vi "StepMotorStateMachine.vi"() -> ()   [LabVIEW 2011]
panel:
  in  "y":i32=360
  out "x-y*floor(x/y)":i32=173
  out "floor(x/y)":i32=148
  out "Diagrama Fasorial":picture
  out "Gauge":dbl(knob)=173.0 scale=0.0..360.0
  out "Counter":i32=53453
  in  "Direccion de Giro":bool=TRUE
  in  "stop":bool
  out "Array":bool[](array[boolean])=[TRUE, FALSE, TRUE, FALSE]
  out "Boolean array":bool[](array[boolean])=[FALSE, TRUE, FALSE, TRUE, FALSE, FALSE, FALSE, FALSE, FALSE, FALSE, FALSE, FALSE, FALSE, FALSE, FALSE, FALSE, FALSE, FALSE, FALSE, FALSE, FALSE, FALSE, FALSE, FALSE, FALSE, FALSE, FALSE, FALSE, FALSE, FALSE, FALSE, FALSE]
  out "Estado":u8=10
  in  "millisecond multiple 2":u32(knob) scale=0.0..300.0
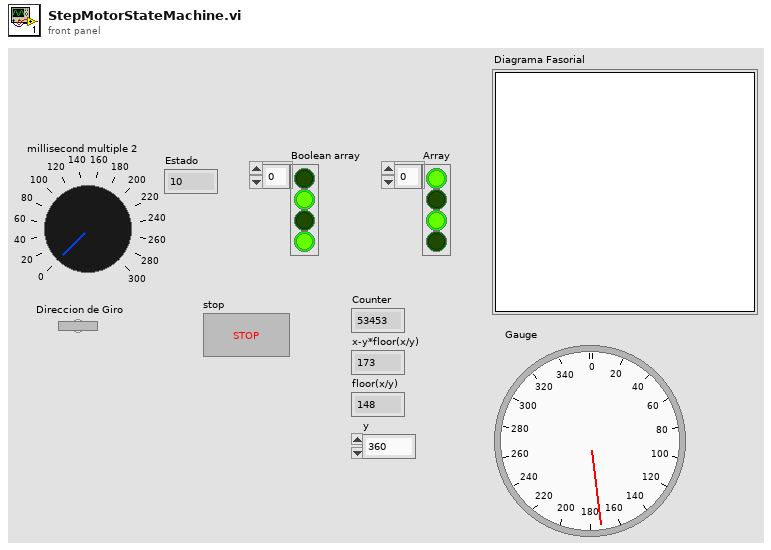
[diagram p1: front panel]
types:
  T1 = typedef "LVBoundsTypeDef.ctl" = cluster{"Width":u32, "Height":u32}
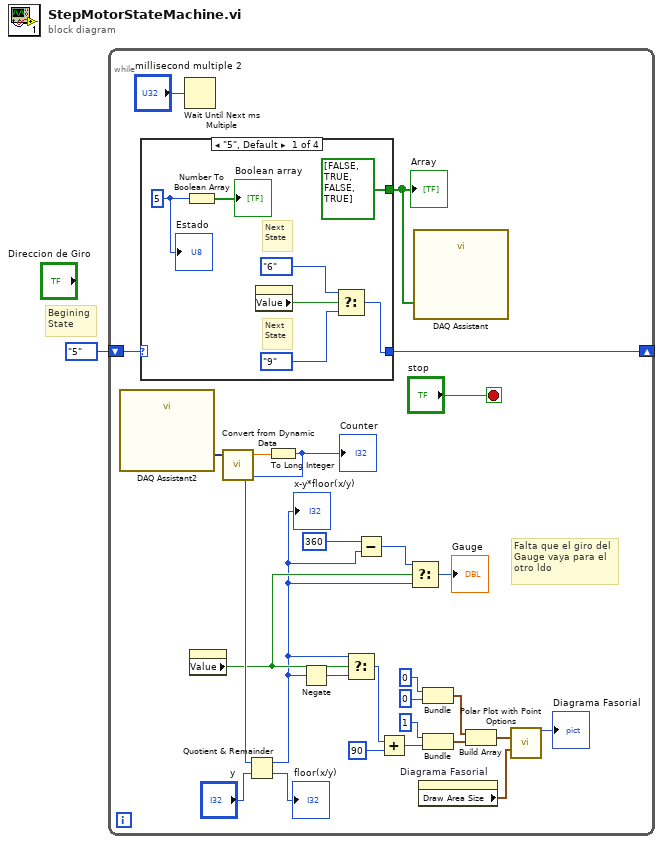
[diagram p0: block diagram]
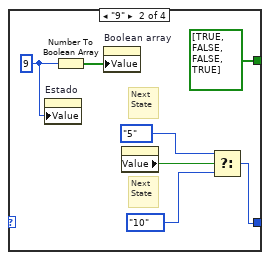
[diagram p2: hidden frame]
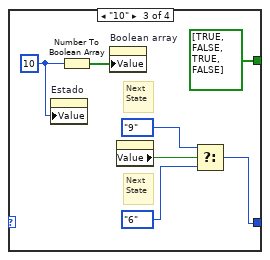
[diagram p3: hidden frame]
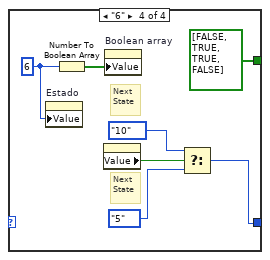
[diagram p4: hidden frame]
diagram:
  # "Begining\nState"
  n1 = while {
    shift-right: [w27] -> _
    shift-left: enum16{"5", "9", "10", "6"}."5" -> [w28]
    stop <- "stop" stop-if-true
    # "Falta que el giro del\nGauge vaya para el\notro ldo"
    n2 = call "DAQ Assistant2"() -> ("data"=w11:dynamicdata)  [unwired: 16 in, 3 out]
    n3 = case shown="\"5\", Default" w28 {
      tunnel: [bool[] [FALSE, TRUE, FALSE, TRUE] bool[] [TRUE, FALSE, FALSE, TRUE] bool[] [TRUE, FALSE, TRUE, FALSE] bool[] [FALSE, TRUE, TRUE, FALSE]] -> w25
      tunnel: [w29 w36 w43 w50] -> w27
      frame "5", Default {
        w35 = 5
        # "Next\nState"
        # "Next\nState"
        n4 = Number To Boolean Array(number=w35) -> (Boolean array=→"Boolean array":bool[])
        n5 = property on="Direccion de Giro" class="Bool (strict)"() -> ("Value"=w30:bool)  [unwired: 2 in, 2 out]
        n6 = Select(t=enum16{"5", "9", "10", "6"}."6", s=w30, f=enum16{"5", "9", "10", "6"}."9") -> (s? t:f=w29:enum16{"5", "9", "10", "6"})
        "Estado" <- w35
      }
      frame "9" {
        w41 = 9
        # "Next\nState"
        # "Next\nState"
        n7 = property on="Estado" class="DigNum (strict)"("Value"=w41) -> ()  [unwired: 2 in, 2 out]
        n8 = Number To Boolean Array(number=w41) -> (Boolean array=w42:bool[])
        n9 = property on="Boolean array" class="Arr (strict)"("Value"=w42) -> ()  [unwired: 2 in, 2 out]
        n10 = property on="Direccion de Giro" class="Bool (strict)"() -> ("Value"=w39:bool)  [unwired: 2 in, 2 out]
        n11 = Select(t=enum16{"5", "9", "10", "6"}."5", s=w39, f=enum16{"5", "9", "10", "6"}."10") -> (s? t:f=w36:enum16{"5", "9", "10", "6"})
      }
      frame "10" {
        w48 = 10
        # "Next\nState"
        # "Next\nState"
        n12 = property on="Estado" class="DigNum (strict)"("Value"=w48) -> ()  [unwired: 2 in, 2 out]
        n13 = Number To Boolean Array(number=w48) -> (Boolean array=w49:bool[])
        n14 = property on="Boolean array" class="Arr (strict)"("Value"=w49) -> ()  [unwired: 2 in, 2 out]
        n15 = property on="Direccion de Giro" class="Bool (strict)"() -> ("Value"=w46:bool)  [unwired: 2 in, 2 out]
        n16 = Select(t=enum16{"5", "9", "10", "6"}."9", s=w46, f=enum16{"5", "9", "10", "6"}."6") -> (s? t:f=w43:enum16{"5", "9", "10", "6"})
      }
      frame "6" {
        w55 = 6
        # "Next\nState"
        # "Next\nState"
        n17 = property on="Estado" class="DigNum (strict)"("Value"=w55) -> ()  [unwired: 2 in, 2 out]
        n18 = Number To Boolean Array(number=w55) -> (Boolean array=w56:bool[])
        n19 = property on="Direccion de Giro" class="Bool (strict)"() -> ("Value"=w53:bool)  [unwired: 2 in, 2 out]
        n20 = property on="Boolean array" class="Arr (strict)"("Value"=w56) -> ()  [unwired: 2 in, 2 out]
        n21 = Select(t=enum16{"5", "9", "10", "6"}."10", s=w53, f=enum16{"5", "9", "10", "6"}."5") -> (s? t:f=w50:enum16{"5", "9", "10", "6"})
      }
    }
    "Array" <- w25
    n22 = Wait Until Next ms Multiple(millisecond multiple="millisecond multiple 2") -> ()  [unwired: 1 out]
    n23 = property on="Direccion de Giro" class="Bool (strict)"() -> ("Value"=w5:bool)  [unwired: 2 in, 2 out]
    n24 = call "Convert from Dynamic Data"("Dynamic Data Type"=w11) -> ("Scalar"=w10:dbl)  [unwired: 3 in]
    n25 = To Long Integer(number=w10) -> (32bit integer=w9:i32)
    "Counter" <- w9
    n26 = Quotient & Remainder(x=w9, y="y") -> (x-y*floor(x/y)=w2:i32, floor(x/y)=→"floor(x/y)":i32)
    "x-y*floor(x/y)" <- w2
    n27 = Negate(x=w2) -> (-x=w7:i32)
    n28 = Select(t=w2, s=w5, f=w7) -> (s? t:f=w8:i32)
    n29 = Subtract(x=360, y=w2) -> (x-y=w3:i32)
    n30 = Add(x=w8, y=90) -> (x+y=w12:i32)
    n31 = Select(t=w3, s=w5, f=w2) -> (s? t:f=→"Gauge":i32)
    n32 = call "DAQ Assistant"("data"=w25) -> ()  [unwired: 17 in, 2 out]
    n33 = property on="Diagrama Fasorial" class="Pict"() -> ("Draw Area Size"=w20:T1)  [unwired: 2 in, 2 out]
    n34 = Bundle(0, 0) -> (w17:cluster{i32, i32})  [unwired: 1 in]
    n35 = Bundle(1, w12) -> (w14:cluster{i32, i32})  [unwired: 1 in]
    n36 = Build Array(w17, w14) -> (w16:cluster{i32, i32}[])
    n37 = call <vilib>:"Polar Plot with Point Options.vi"("data array [mag, phase (deg)]"=w16, "dimensions (w,h)"=w20) -> ("new picture"=→"Diagrama Fasorial":picture)  [unwired: 13 in]
  }
